vi "Fetch Waveform.vi"(7 "Waveform Start (1)":i32=1, 8 "error in (no error)":errorcluster {"code" format="%.0x"}, 9 "Waveform End (10000)":i32=10000, 10 "Source (Channel 1)":string(combo)="CH1", 11 "VISA Resource Name":refnum<visa-resource-name>) -> (0 "error out":errorcluster {"code" format="%.0x"}, 1 "X Increment":dbl format="%.2e", 2 "Initial X":dbl format="%.2e", 3 "VISA Resource Name Out":refnum<visa-resource-name>, 4 "Waveform Array":dbl[](array[numeric]) format="%.2f", 5 "Actual Points":u32)   [LabVIEW 2010, in "Tektronix TDS 3000 Series.lvlib"]
doc: "This VI reads the current waveform (starting and ending at Waveform Start and Waveform End,respectively) from the oscilloscope, scales the data, and returns an array of DBLs. To obtain the complete waveform, use the default values on the waveform start and waveform end controls.\n\nNote:\n(1) In order for this VI to work the waveform must be displayed on the instrument.\n(2) This is only used with Normal and Average Acquisition Types\n(3) The instrument will return an error if you attempt to read more points than stored on the instrument. Set the desired record length in the Configure Acquisition Record VI."
uses:
  <instrlib>/Tektronix TDS 3000 Series/Tektronix TDS 3000 Series.lvlib
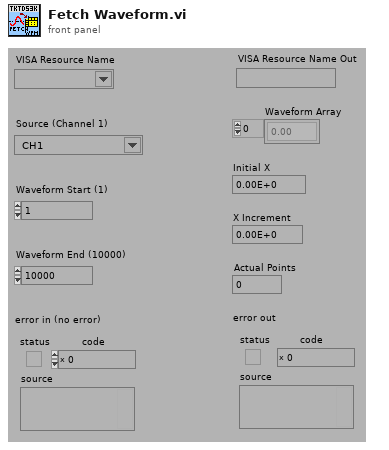
[diagram p1: front panel]
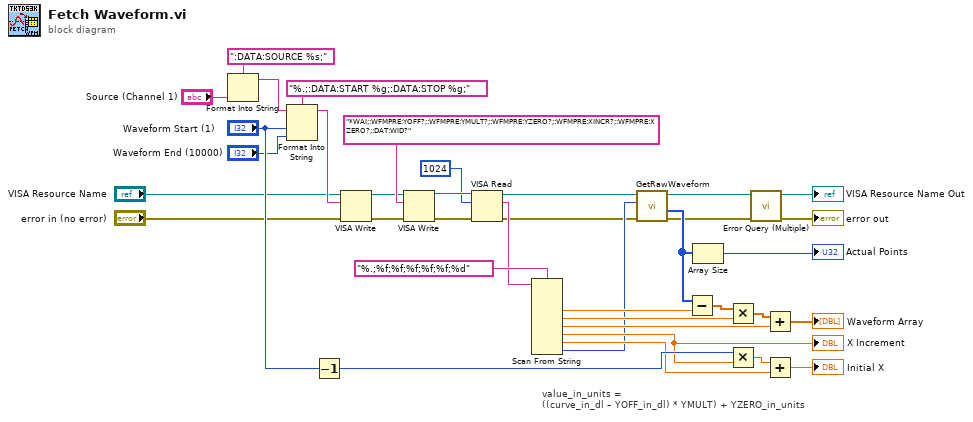
[diagram p0: block diagram]
diagram:
  # "value_in_units =\n((curve_in_dl – YOFF_in_dl) * YMULT) + YZERO_in_units"
  n1 = Format Into String(format string=":DATA:SOURCE %s;", "Source (Channel 1)") -> (resulting string=w34:string)  [unwired: 2 in, 1 out]
  n2 = Format Into String(format string="%.;:DATA:START %g;:DATA:STOP %g;", initial string=w34, "Waveform Start (1)", "Waveform End (10000)") -> (resulting string=w14:string)  [unwired: 1 in, 1 out]
  n3 = Decrement(x="Waveform Start (1)") -> (x-1=w20:i32)
  n4 = VISA Write(VISA resource name="VISA Resource Name", write buffer=w14, error in (no error)="error in (no error)") -> (VISA resource name out=w28:refnum<visa-resource-name>, error out=w27:errorcluster)  [unwired: 1 out]
  n5 = VISA Write(VISA resource name=w28, write buffer="*WAI;:WFMPRE:YOFF?;:WFMPRE:YMULT?;:WFMPRE:YZERO?;:WFMPRE:XINCR?;:WFMPRE:XZERO?;:DAT:WID?", error in (no error)=w27) -> (VISA resource name out=w32:refnum<visa-resource-name>, error out=w33:errorcluster)  [unwired: 1 out]
  n6 = VISA Read(VISA resource name=w32, byte count=u32 1024 ("byte count (0)"), error in (no error)=w33) -> (VISA resource name out=w5:refnum<visa-resource-name>, read buffer=w29:string, error out=w6:errorcluster)  [unwired: 1 out]
  n7 = Scan From String(format string="%.;%f;%f;%f;%f;%f;%d", input string=w29) -> (output 1=w24:dbl, output 2=w22:dbl, output 3=w21:dbl, output 4=w17:dbl, output 5=w18:dbl, output 6=w7:i32)  [unwired: 8 in, 3 out]
  "X Increment" <- w17
  n8 = call <instrlib>:"GetRawWaveform.vi"("error in (no error)"=w6, "Byte Size per point (1 byte)"=w7, "VISA Resource Name"=w5) -> ("error out"=w3:errorcluster, "Waveform Array"=w8:i16[], "VISA Resource Name Out"=w4:refnum<visa-resource-name>)  [unwired: 6 in]
  n9 = Subtract(x=w8, y=w24) -> (x-y=w23:dbl[])
  n10 = Array Size(array=w8) -> (size(s)=→"Actual Points":i32)
  n11 = Multiply(x=w23, y=w22) -> (x*y=w26:dbl[])
  n12 = Multiply(x=w20, y=w17) -> (x*y=w19:dbl)
  n13 = call <instrlib>:"Error Query (Multiple).vi"("error in (no error)"=w3, "VISA Resource Name"=w4) -> ("error out"=→"error out":errorcluster, "VISA Resource Name Out"=→"VISA Resource Name Out":refnum<visa-resource-name>)  [unwired: 6 in, 2 out]
  n14 = Add(x=w26, y=w21) -> (x+y=→"Waveform Array":dbl[])
  n15 = Add(x=w19, y=w18) -> (x+y=→"Initial X":dbl)
